vi "Robot1.vi"() -> ()   [LabVIEW 2011]
uses:
  <vilib>/NXT/Subs/MotorOutput.ctl
  <vilib>/NXT/Block Support/NXT_InputPort.ctl
  <vilib>/NXT/Dual Mode Library/Sensors/Sound_dB.vi
  <vilib>/NXT/Dual Mode Library/Sensors/Sonar_cm.vi
  <vilib>/NXT/Dual Mode Library/Sensors/Touch_Pressed.vi
  <vilib>/NXT/Dual Mode Library/Sensors/Light_On.vi
  <vilib>/NXT/Dual Mode Library/Motors/MotorReverse.vi
  <vilib>/NXT/Dual Mode Library/Motors/MotorOn.vi
panel:
  out "Miic: Sound (dB)":i16(graph) caption="Sound (dB)"
  out "Light: Scaled Value":i16(graph) caption="Scaled Value"
  out "Sonar: Distance (cm)":i16(graph) caption="Distance (cm)"
  out "Yes / No":bool caption="Touch: Yes / No"
  in  "stop":bool
  in  "F speed (0-75)":i32(knob)=75 scale=0.0..75.0
  in  "F Motor Port":T1=6 items=["Port A"=0, "Port B"=1, "Port C"=2, "Ports A & B"=4, "Ports A & C"=5, "Ports B & C"=6, "All Ports"=3]
  in  "B speed (0-75)":i32(knob)=75 scale=0.0..75.0
  in  "R Motor Port":T1=3 items=["Port A"=0, "Port B"=1, "Port C"=2, "Ports A & B"=4, "Ports A & C"=5, "Ports B & C"=6, "All Ports"=3]
  in  "Direction":bool
  # "LEGO MINDSTORM CONTROL AND INDICATOR PANEL"
  # "Robot Sensors/Indicators"
  # "Robot Controls"
  # "SERIAL # MCGILLDBE13032010:  MADE IN  CANADA: © NANDKISHOR M. DHAWALE / VIACHESLAV  I. ADAMCHUK"
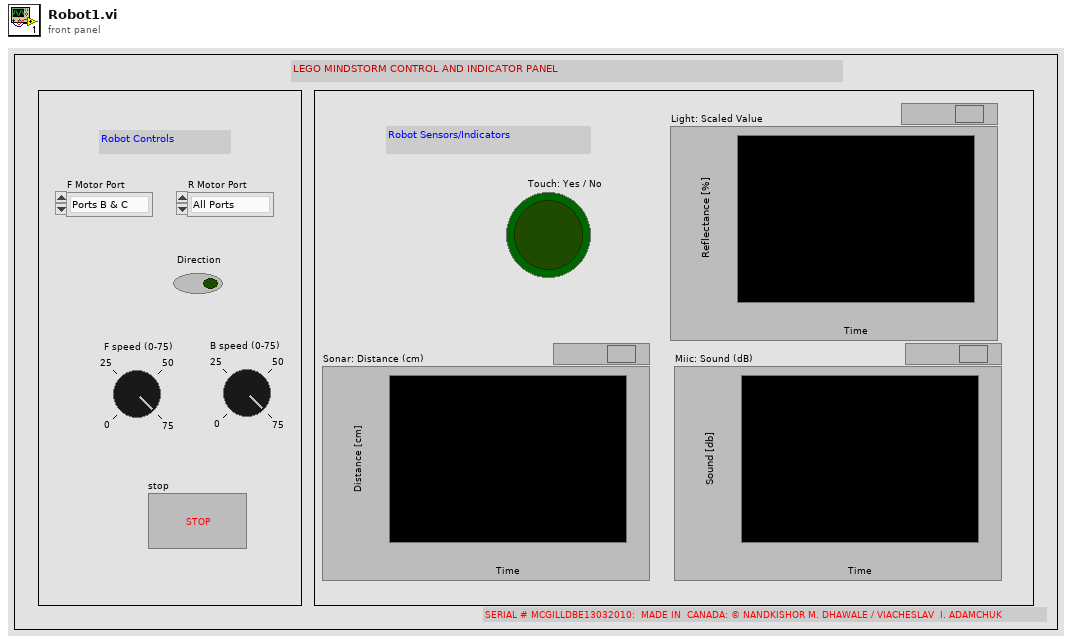
[diagram p1: front panel]
types:
  T1 = typedef "MotorOutput.ctl" = u8
  T2 = typedef "NXT_InputPort.ctl" = u8
  T3 = typedef "LVHSConnector.ctl" = cluster{"Hardware":string, "Flattened String":string}
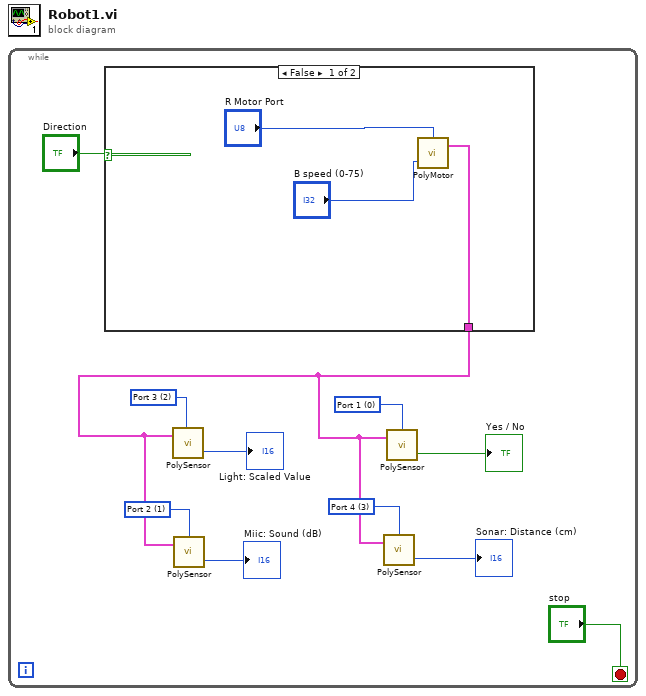
[diagram p0: block diagram]
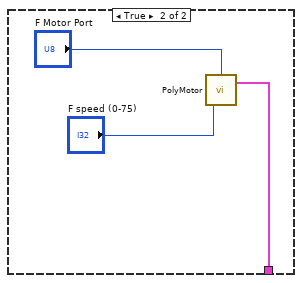
[diagram p2: hidden frame]
diagram:
  n1 = while {
    stop <- "stop" stop-if-true
    w5 = T2 3 items=["Port 1", "Port 2", "Port 3", "Port 4"] ("Port (Port 4)")
    w4 = T2 1 items=["Port 1", "Port 2", "Port 3", "Port 4"] ("Port (Port 2)")
    w3 = T2 0 items=["Port 1", "Port 2", "Port 3", "Port 4"] ("Port (Port 1)")
    w2 = T2 2 items=["Port 1", "Port 2", "Port 3", "Port 4"] ("Port (Port 3)")
    n2 = case shown="False" "Direction" {
      tunnel: [w12 w15] -> w1
      frame False {
        n3 = call-poly <vilib>:"PolyMotor.vi"("Power (75)"="B speed (0-75)", "Output Port (All Ports)"="R Motor Port") -> ("NXT"=w12:T3)  [unwired: 2 in]
      }
      frame True {
        n4 = call-poly <vilib>:"PolyMotor.vi"("Power (75)"="F speed (0-75)", "Output Port (All Ports)"="F Motor Port") -> ("NXT"=w15:T3)  [unwired: 2 in]
      }
    }
    n5 = call-poly <vilib>:"PolySensor.vi"("NXT"=w1, "Port (Port 3)"=w2) -> ("Scaled Value"=→"Light: Scaled Value":i16)  [unwired: 1 in, 1 out]
    n6 = call-poly <vilib>:"PolySensor.vi"("NXT"=w1, "Port (Port 2)"=w4) -> ("Sound (dB)"=→"Miic: Sound (dB)":i16)  [unwired: 1 in, 1 out]
    n7 = call-poly <vilib>:"PolySensor.vi"("NXT"=w1, "Port (Port 4)"=w5) -> ("Distance (cm)"=→"Sonar: Distance (cm)":i16)  [unwired: 1 in, 1 out]
    n8 = call-poly <vilib>:"PolySensor.vi"("NXT"=w1, "Port (Port 1)"=w3) -> ("Yes / No"=→"Yes / No":bool)  [unwired: 1 in, 1 out]
  }
